vi "gen_sine_shift.vi"(4 "Filter Cluster":T1={"Ditigal Low pass?"=FALSE, "Max Freq"=20.0} {"Max Freq" format="%#_13g"}, 5 "TxRxParams":T2={"sample rate"=1000000.0, "Transmit frequency"=25000.0, "Transmit amplitude"=1.577, "sample rate digital out"=40000.0, "TX cycles"=600, "sample rate DAQ1"=1000000.0, "Receive frequency"=75000.0, "Receive range"=1.0, "TX harmonics"=[50000.0, 75000.0, 100000.0, 125000.0, 150000.0, 175000.0, 200000.0, 225000.0]} {"TX harmonics" format="%#_6p"; "Receive frequency" format="%#_6p"; "sample rate DAQ1" format="%#_6p"; "sample rate digital out" format="%#_6p"; "Transmit frequency" format="%#_6p"; "sample rate" format="%#_6p"}, 6 "signal type":T3(ring)=enum."Triangle Wave", 7 "no of TX cycles per image":dbl=60000.0, 8 "Shift DC offset":dbl, 9 "Shift Amplitude (pk)":dbl=1.0, 10 "time lag of shift system":dbl=0.2 format="%.2p", 11 "no of TX cycles per shift cycle":dbl=12000.0) -> (0 "signal out":waveform(dbl), 3 "Shift frequency":dbl=2.0833333333333335)   [LabVIEW 2021]
uses:
  <vilib>/measure/NI_MABase.lvlib
panel:
  out "size(s)":i32
  out "sample rate":dbl=1000000.0 format="%#_6p"
  out "Transmit frequency":dbl=25000.0 format="%#_6p"
  out "phase offset (deg)":dbl=150.00000000000003
  out "Waveform Graph":waveform(dbl)(graph)={"t0"=timestamp(0 s since 1904-01-01), "dt"=1e-06, "Y"=array[240000 elements]}
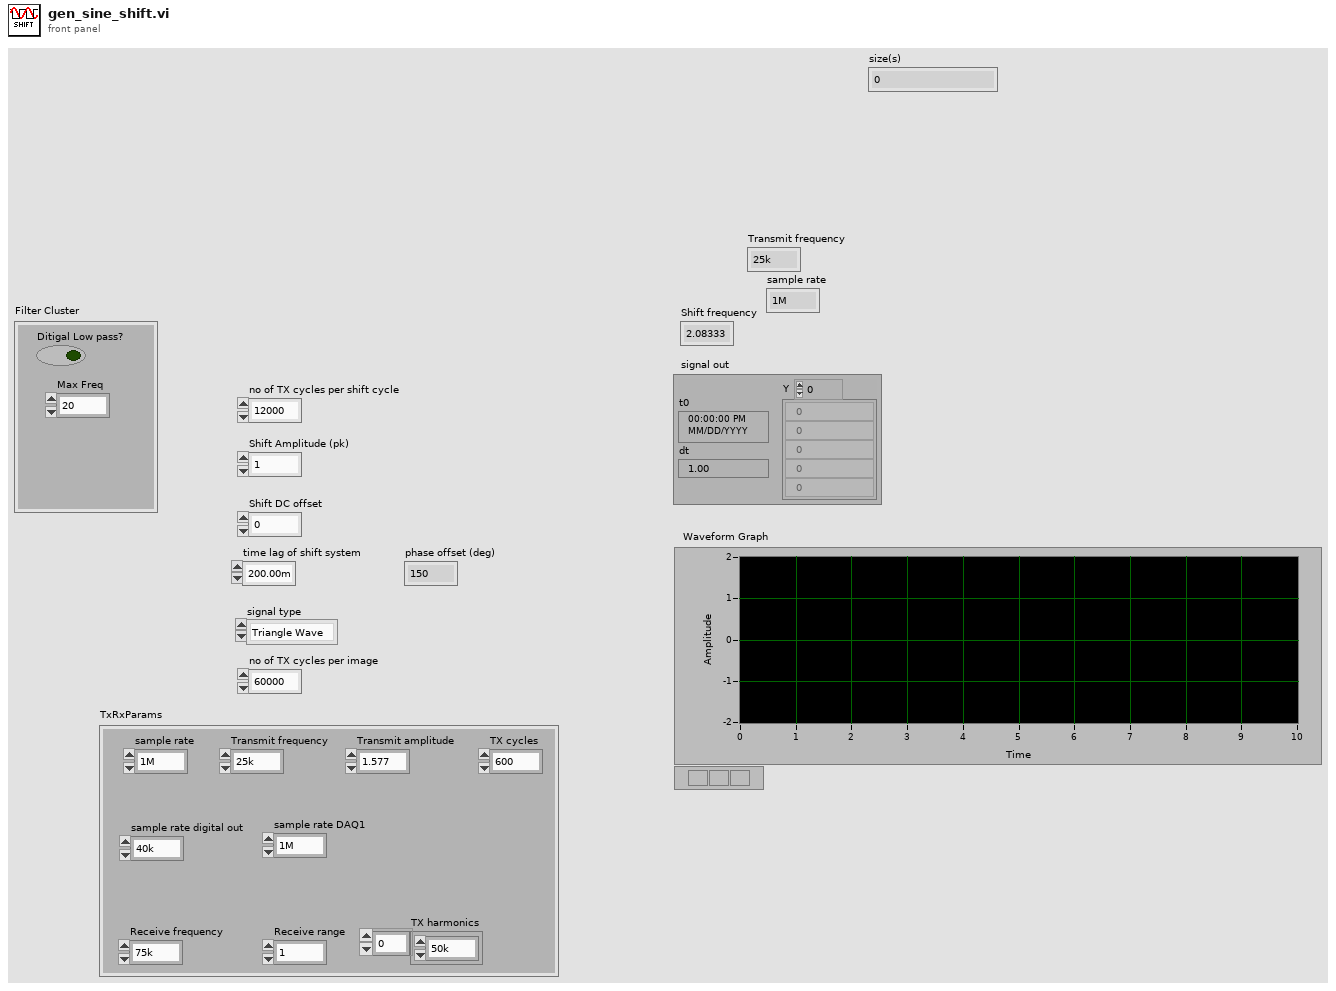
[diagram p1: front panel]
types:
  T1 = cluster{"Ditigal Low pass?":bool, "Max Freq":dbl}
  T2 = cluster{"sample rate":dbl, "Transmit frequency":dbl, "Transmit amplitude":dbl, "sample rate digital out":dbl, "TX cycles":i32, "sample rate DAQ1":dbl, "Receive frequency":dbl, "Receive range":dbl, "TX harmonics":dbl[]}
  T3 = enum16{"Sine Wave", "Triangle Wave", "Square Wave", "Sawtooth Wave"}
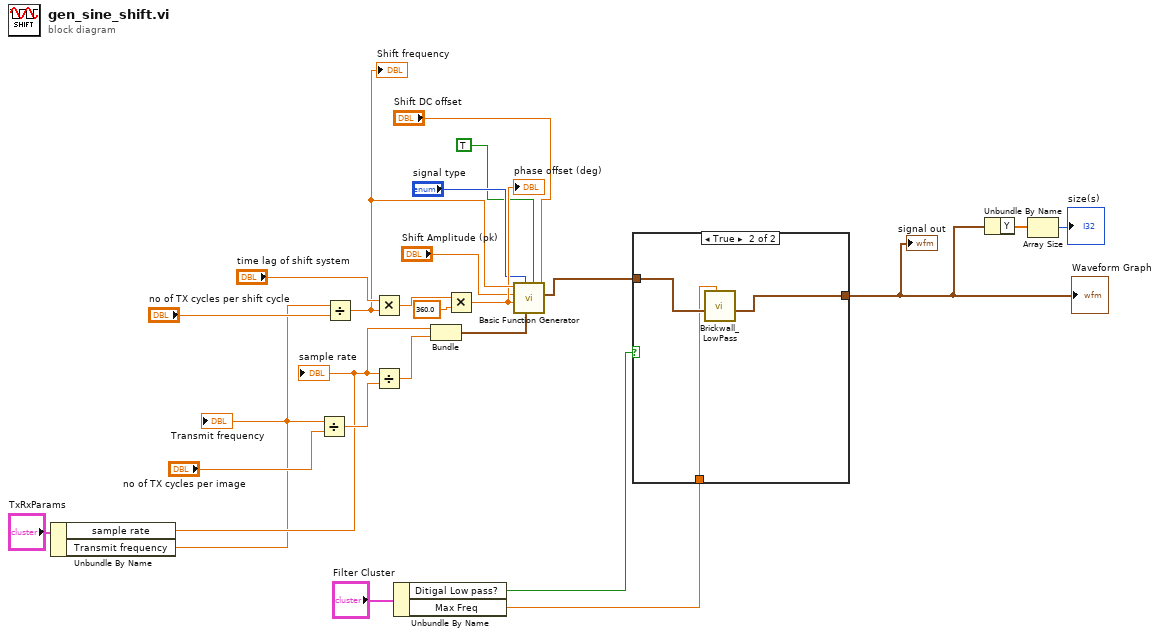
[diagram p0: block diagram]
diagram:
  n1 = Unbundle By Name("TxRxParams") -> ("sample rate"=w9:dbl, "Transmit frequency"=w8:dbl)
  "Transmit frequency" <- w8
  "sample rate" <- w9
  n2 = Divide(x=w8, y="no of TX cycles per image") -> (x/y=w13:dbl)
  n3 = Divide(x=w8, y="no of TX cycles per shift cycle") -> (x/y=w20:dbl)
  "Shift frequency" <- w20
  n4 = Multiply(x="time lag of shift system", y=w20) -> (x*y=w19:dbl)
  n5 = Divide(x=w9, y=w13) -> (x/y=w23:dbl)
  n6 = Unbundle By Name("Filter Cluster") -> ("Ditigal Low pass?"=w5:bool, "Max Freq"=w4:dbl)
  n7 = Bundle("sample rate"=w9, w23) -> (w24:cluster{"sample rate":dbl, dbl})  [unwired: 1 in]
  n8 = Multiply(x=w19, y=360.0) -> (x*y=w17:dbl)
  "phase offset (deg)" <- w17
  n9 = call <vilib>:"Basic Function Generator.vi"("offset"="Shift DC offset", "reset signal"=TRUE, "sampling info"=w24, "signal type"="signal type", "phase"=w17, "amplitude"="Shift Amplitude (pk)", "frequency"=w20) -> ("signal out"=w7:waveform(dbl))  [unwired: 2 in, 2 out]
  n10 = case shown="True" w5 {
    tunnel: w7 -> [w25 w28]
    tunnel: [w25 w27] -> w3
    tunnel: w4 -> [_ w26]
    frame False {
    }
    frame True {
      n11 = call "Brickwall_LowPass.vi"("Max Freq"=w26, "time signal"=w28) -> ("output waveform"=w27:waveform(dbl))  [unwired: 5 in, 4 out]
    }
  }
  "signal out" <- w3
  "Waveform Graph" <- w3
  n12 = Unbundle By Name(w3) -> ("Y"=w2:dbl[])
  n13 = Array Size(array=w2) -> (size(s)=→"size(s)":i32)
